vi "FIR Narrowband Filter (CDB).vi"(2 "IFIR Coefficients":T1 {"Image Suppressor" format="%0.2e"; "Model Filter" format="%0.2e"}, 3 "X":cdb[](array[numeric])) -> (0 "error":i32, 1 "Filtered X":cdb[](array[numeric]))   [LabVIEW 2014, in "NI_AALBase.lvlib"]
doc: "Filters the input sequence <B>X</B> using the interpolated FIR (IFIR) filter specified by <B>IFIR Coefficients</B>."
uses:
  NI_AALBase.lvlib
  lvanlys.dll
panel:
  # "FIR Narrowband Filter"
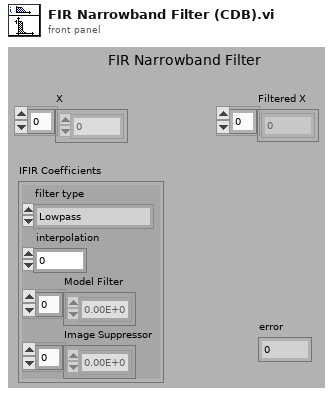
[diagram p1: front panel]
types:
  T1 = cluster{"filter type":enum32{"Lowpass", "Highpass", "Bandpass", "Bandstop", "Wideband-Lowpass", "Wideband-Highpass"}, "interpolation":i32, "Model Filter":dbl[], "Image Suppressor":dbl[]}
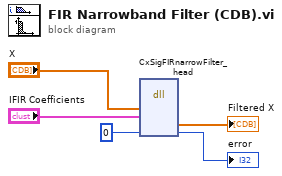
[diagram p0: block diagram]
diagram:
  n1 = dll-call lib="C:/Program Files (x86)/National Instruments/LabVIEW 2014/resource/lvanlys.*" fn="CxSigFIRnarrowFilter_head"("xH"="X", "coefC"="IFIR Coefficients", "dsperr"=0) -> ("Filtered X"=→"Filtered X":cdb[], "dsperr"=→"error":i32)  [unwired: 5 in, 4 out]
